vi "Durability Endpoints Calc.vi"(10 "Data Cluster":T2, 11 "Configuration Data in":T1) -> (1 "Target RIght Position":dbl, 2 "Target Left Position":dbl, 3 "Configuration Data out":T1)   [LabVIEW 2026, in "Acquisition.lvlib"]
uses:
  Acquisition.lvlib
  Hardware Configuration.ctl
  controls/Test Config Data.ctl
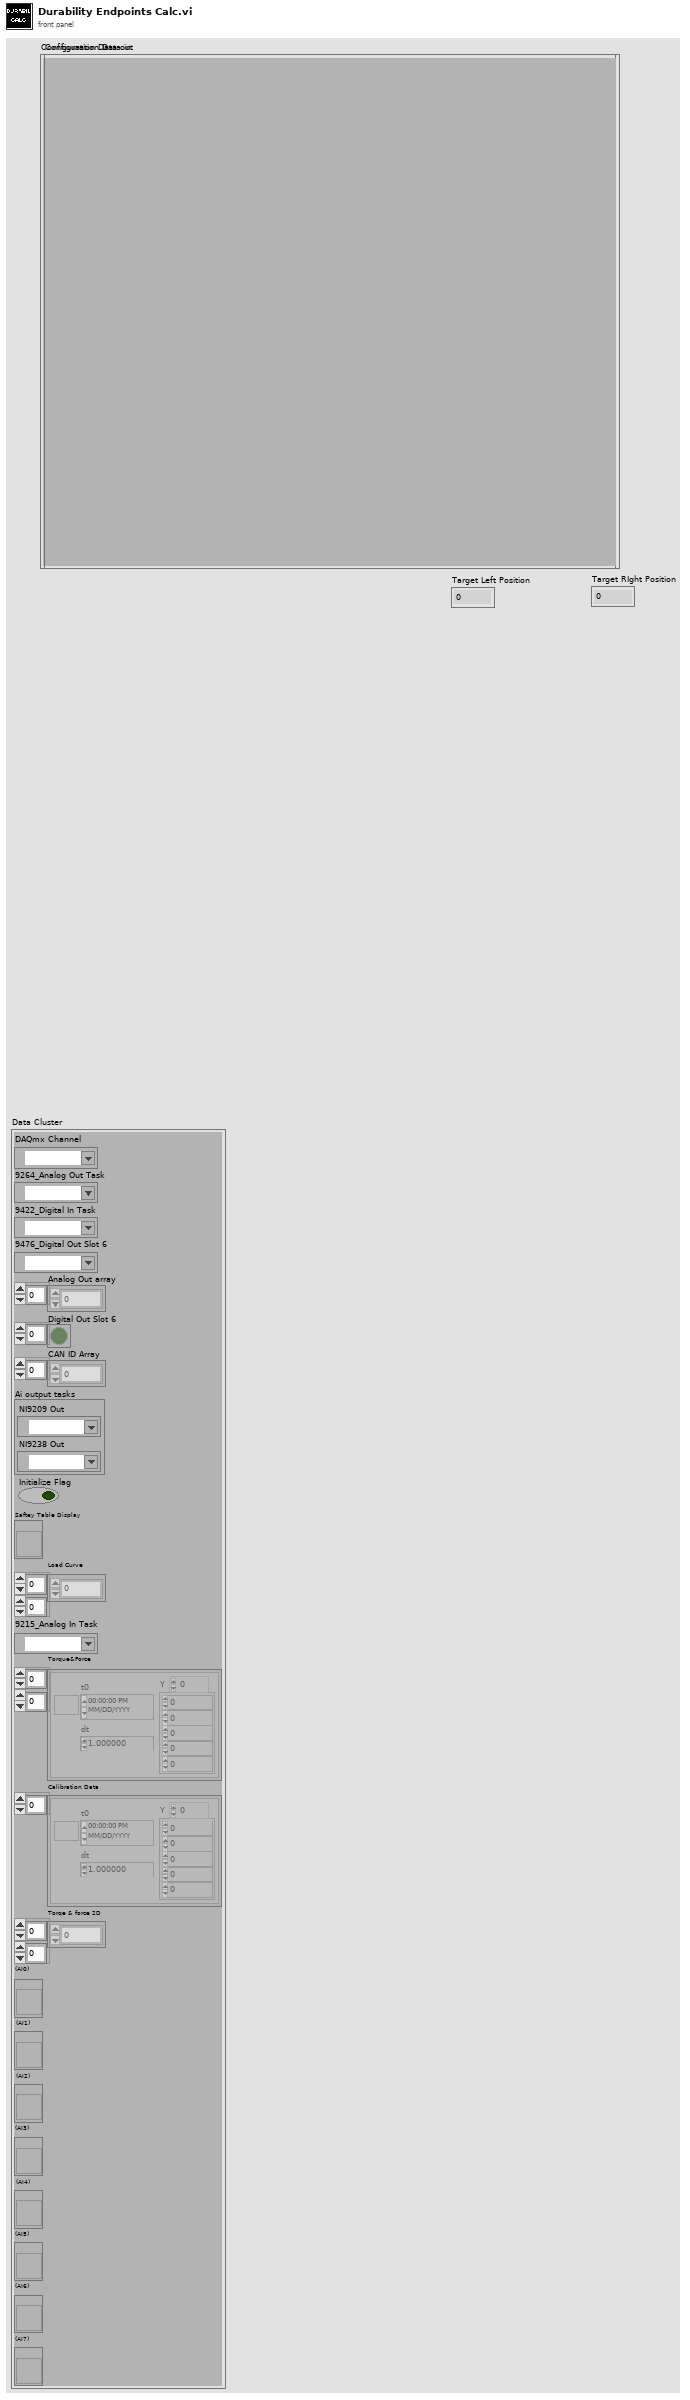
[diagram p1: front panel]
types:
  T1 = typedef "Test Config Data.ctl" = cluster{}
  T2 = typedef "Acquisition.lvlib/Hardware Configuration.ctl" = cluster{"DAQmx Channel":tag, "9264_Analog Out Task":refnum<k21>, "9422_Digital In Task":refnum<k21>, "9476_Digital Out Slot 6":refnum<k21>, "Analog Out array":dbl[], "Digital Out Slot 6":bool[], "CAN ID Array":u32[], "Ai output tasks":cluster{"NI9209 Out":refnum<k21>, "NI9238 Out":refnum<k21>}, "Initialize Flag":bool, "Saftey Table Display":refnum<vi>, "Load Curve":dbl[][], "9215_Analog In Task":refnum<k21>, "Torque&Force":waveform(dbl)[][], "Calibration Data":waveform(dbl)[], "Torqe & force 2D":dbl[][], "(AI0)":refnum<vi>, "(AI1)":refnum<vi>, "(AI2)":refnum<vi>, "(AI3)":refnum<vi>, "(AI4)":refnum<vi>, "(AI5)":refnum<vi>, "(AI6)":refnum<vi>, "(AI7)":refnum<vi>}
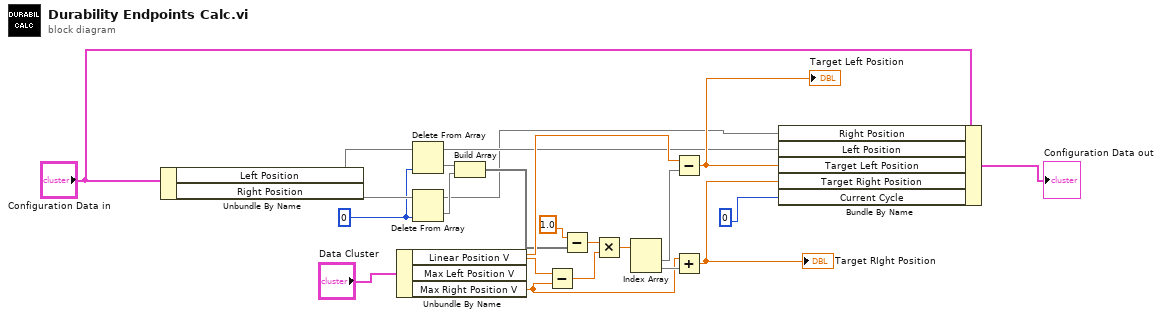
[diagram p0: block diagram]
diagram:
  w3 = 0 ("index")
  n1 = Unbundle By Name("Configuration Data in") -> ("Left Position"=w7, "Right Position"=w4)
  n2 = Unbundle By Name("Data Cluster") -> ("Max Left Position V"=w13:dbl, "Max Right Position V"=w15:dbl)  [unwired: 1 out]
  n3 = Delete From Array(array=w7, index=w3) -> (deleted portion=w6, array with subset deleted=w2)  [unwired: 1 in]
  n4 = Delete From Array(array=w4, index=w3) -> (deleted portion=w5, array with subset deleted=w1)  [unwired: 1 in]
  n5 = Build Array(w6, w5) -> (w8:void[])
  n6 = Subtract(x=w13, y=w15) -> (x-y=w9:dbl)
  n7 = Subtract(x=1.0, y=w8) -> (x-y=w12:dbl)
  n8 = Multiply(x=w12, y=w9) -> (x*y=w10:dbl)
  n9 = Index Array(array=w10) -> (element #1=w14, element #2=w16)  [unwired: 2 in]
  n10 = Subtract(x=w13, y=w14) -> (x-y=w19:dbl)
  "Target Left Position" <- w19
  n11 = Add(x=w15, y=w16) -> (x+y=w20:dbl)
  "Target RIght Position" <- w20
  n12 = Bundle By Name(cluster="Configuration Data in", "Right Position"=w1, "Left Position"=w2, "Target Left Position"=w19, "Target Right Position"=w20, "Current Cycle"=u64 0) -> (→"Configuration Data out":T1)
